vi "CRYRecall Curve Name Replace.vi"(6 "Data type":string, 7 "Setup in":T1={"No.VI"=0, "Category"="", "StepName"="", "Seq setup flattened"="", "Comment"="", "Steps config."=[], "Jump config"=[], "Start"=0.0, "Increment"=0.0, "Name"="Pa", "Unit"="Pa", "Y data"=1, "Y prefix"="", "Y dB ref"=1.0, "Y unit"="", "Repeat State Array"=[]} {"Repeat State Array"."Start" format="%#_5g"; "Y dB ref" format="%.1f"; "Y data" items=["dB", "Lin"]; "Start" format="%#_5g"}, 9 "Step setup In":string, 11 "sOption1":string="SameRemain") -> ()   [LabVIEW 2013]
uses:
  Typedef Control/CRYStep.ctl
  Typedef Control/CRYResult Cluster Array.ctl
  Typedef Control/CRYResult Cluster.ctl
  Typedef Control/CRYData Cluster Array.ctl
  Typedef Control/CRYData Cluster.ctl
  Typedef Control/CRYWaveform Cluster Array.ctl
  Typedef Control/CRYWaveform Cluster.ctl
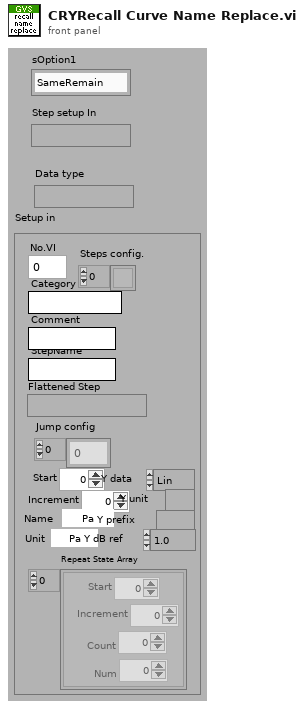
[diagram p1: front panel]
types:
  T1 = typedef "CRYStep.ctl" = cluster{"No.VI":i32, "Category":string, "StepName":string, "Seq setup flattened":string, "Comment":string, "Steps config.":bool[], "Jump config":i32[], "Start":dbl, "Increment":dbl, "Name":string, "Unit":string, "Y data":u16, "Y prefix":string, "Y dB ref":dbl, "Y unit":string, "Repeat State Array":cluster{"Start":dbl, "Increment":dbl, "Count":i32, "Num":i32}[]}
  T2 = typedef "CRYWaveform Cluster Array.ctl" = T3[]
  T3 = typedef "CRYWaveform Cluster.ctl" = cluster{"Waveform":cluster{"X0":dbl, "dX":dbl, "Y":sgl[]}, "X data":u16, "Y data":u16, "Y axis":u16, "X unit":string, "Y unit":string, "Y dB ref":dbl, "display Y":bool, "display X":bool, "Overload?":bool, "Test Info":string, "Step No.":i32, "Name":string, "protected":bool, "Sqc history":string[], "Signal Channel ID":i32, "Plot Settings":cluster{"Color":u32, "Interpolation":u8, "Point Style":u8, "Line Style":u8, "Point Color":u32, "Line Width":u8, "Bar Plot Style":u8, "Fill To":i16}, "AutoProtect":bool}
  T4 = typedef "CRYData Cluster Array.ctl" = T5[]
  T5 = typedef "CRYData Cluster.ctl" = cluster{"Name":string, "Curve":cluster{"x":dbl, "y":dbl, "z":dbl}[], "X data":u16, "Y data":u16, "Z data":u16, "X axis":u16, "Y axis":u16, "Z axis":u16, "X unit":string, "Y unit":string, "Z unit":string, "X dB ref":dbl, "Y dB ref":dbl, "Z dB ref":dbl, "single val":bool, "protected":bool, "display X":bool, "display Y":bool, "display Z":bool, "Test Info":string, "Step No.":i32, "Plot Settings":cluster{"Color":u32, "Interpolation":u8, "Point Style":u8, "Line Style":u8, "Point Color":u32, "Line Width":u8, "Bar Plot Style":u8, "Fill To":i16}, "AutoProtect":bool}
  T6 = typedef "CRYResult Cluster Array.ctl" = T7[]
  T7 = typedef "CRYResult Cluster.ctl" = cluster{"Name":string, "Margin":dbl, "unit":string, "Verdict":bool, "Limit":string, "Max/Min":string, "protected":bool, "Step No.":i32, "Test Info":string, "AutoProtect":bool}
  T8 = cluster{"Start":dbl, "Increment":dbl, "Count":i32, "Num":i32}[]
  T9 = typedef "CRYRecall Cluster.ctl" = cluster{"Name":string, "filepath":string, "all or last":i32, "File Path Mode":u16, "Curve Names":string[], "format string":cluster{"dB Format String out":string, "Lin Format String out":string}, "Template":u16[], "Axis":u16, "*.imp Path":path, "Filepath option":i16, "ML Value":dbl, "user defined":string, "Curves Selected?":bool[], "Help":string, "Tab Value":enum32{"Setting", "Help"}, "Selector":i32, "Use Default":bool}
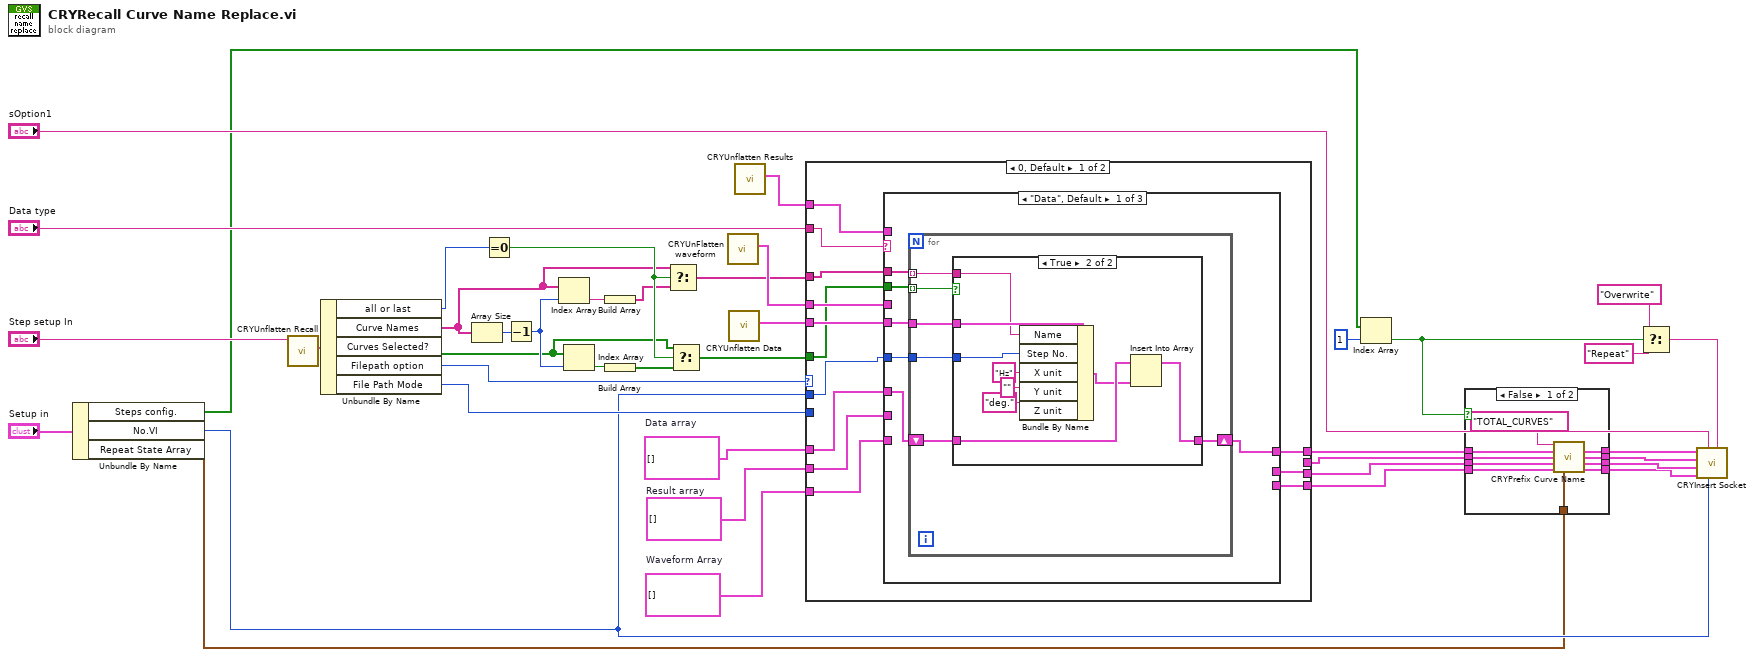
[diagram p0: block diagram]
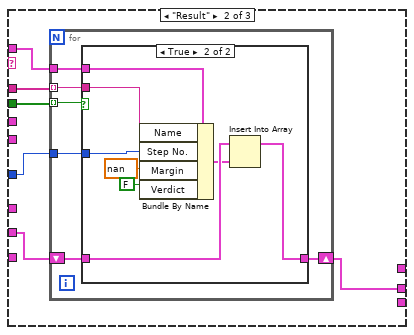
[diagram p4: hidden frame]
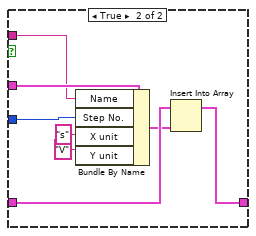
[diagram p7: hidden frame]
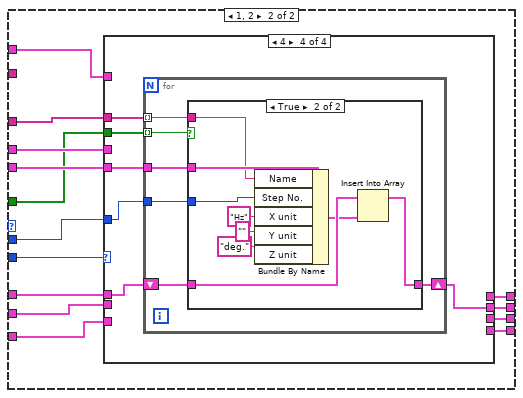
[diagram p8: hidden frame]
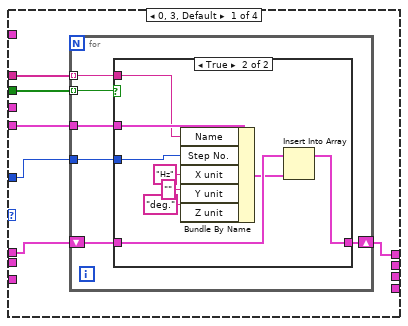
[diagram p9: hidden frame]
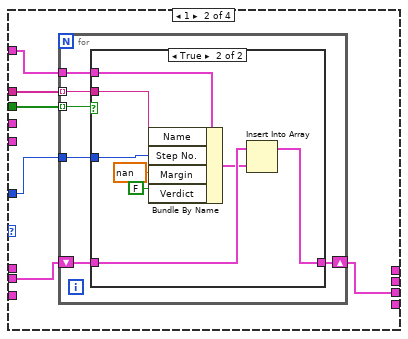
[diagram p11: hidden frame]
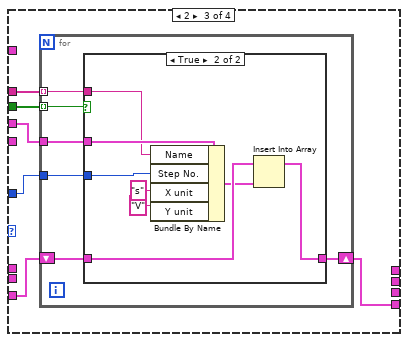
[diagram p13: hidden frame]
diagram:
  w36 = T2 []  # Waveform Array
  w38 = T4 []  # Data array
  w37 = T6 []  # Result array
  n1 = Unbundle By Name("Setup in") -> ("Steps config."=w11:bool[], "No.VI"=w12:i32, "Repeat State Array"=w1:T8)
  n2 = call "CRYUnflatten Recall.vi"("Flatten Recall"="Step setup In") -> ("Recall setup"=w30:T9)  [unwired: 8 in, 2 out]
  n3 = Unbundle By Name(w30) -> ("all or last"=w27:i32, "Curve Names"=w21:string[], "Curves Selected?"=w18:bool[], "Filepath option"=w29:i16, "File Path Mode"=w28:u16)
  n4 = Array Size(array=w21) -> (size(s)=w26:i32)
  n5 = Equal To 0?(x=w27) -> (x = 0?=w22:bool)
  n6 = Decrement(x=w26) -> (x-1=w25:i32)
  n7 = Index Array(array=w21, index=w25) -> (element=w23:string)
  n8 = Index Array(array=w18, index=w25) -> (element=w24:bool)
  n9 = Build Array(w23) -> (w20:string[])
  n10 = Build Array(w24) -> (w19:bool[])
  n11 = Select(t=w21, s=w22, f=w20) -> (s? t:f=w17:string[])
  n12 = Select(t=w18, s=w22, f=w19) -> (s? t:f=w16:bool[])
  n13 = call "CRYUnFlatten waveform.vi"() -> ("Waveform Cluster"=w39:T3)  [unwired: 9 in, 2 out]
  n14 = call "CRYUnflatten Data.vi"() -> ("Datum"=w41:T5)  [unwired: 9 in, 2 out]
  n15 = call "CRYUnflatten Results.vi"() -> ("Result"=w40:T7)  [unwired: 9 in, 2 out]
  n16 = case shown="0, Default" w29 {
    tunnel: w41 -> [w54 w132]
    tunnel: w12 -> [w53 w131]
    tunnel: [w52 w130] -> w10
    tunnel: [_ w129] -> w9
    tunnel: [w50 w128] -> w8
    tunnel: [w49 w127] -> w7
    tunnel: w40 -> [w51 w126]
    tunnel: w39 -> [w48 w125]
    tunnel: w38 -> [w46 w123]
    tunnel: w37 -> [w45 w122]
    tunnel: w36 -> [w47 w124]
    tunnel: w28 -> [_ w121]
    tunnel: w17 -> [w44 w120]
    tunnel: w16 -> [w43 w119]
    tunnel: "Data type" -> [w42 _]
    frame 0, Default {
      n17 = case shown="\"Data\", Default" w42 {
        tunnel: w44 -> [w60 w82 w103]
        tunnel: w43 -> [w59 w81 w102]
        tunnel: w54 -> [w58 _ _]
        tunnel: w53 -> [w57 w79 w100]
        tunnel: w47 -> [_ _ w99]
        tunnel: [w55 _ _] -> w52
        tunnel: w51 -> [_ w80 _]
        tunnel: [_ w78 _] -> w50
        tunnel: [_ _ w98] -> w49
        tunnel: w48 -> [_ _ w101]
        tunnel: w46 -> [w56 _ _]
        tunnel: w45 -> [_ w77 _]
        frame "Data", Default {
          n18 = for {
            tunnel: w60 -> [w66] mode=indexing
            shift-right: [w64] -> w55
            shift-left: w56 -> [w65]
            tunnel: w59 -> [w63] mode=indexing
            tunnel: w58 -> [w62]
            tunnel: w57 -> [w61]
            n19 = case shown="True" w63 {
              tunnel: w66 -> [_ w74]
              tunnel: w65 -> [w67 w70]
              tunnel: [w67 w69] -> w64
              tunnel: w62 -> [_ w76]
              tunnel: w61 -> [_ w75]
              frame False {
              }
              frame True {
                n20 = Bundle By Name(cluster=w76, "Name"=w74, "Step No."=w75, "X unit"="Hz", "Y unit"="", "Z unit"="deg.") -> (w68:T5)
                n21 = Insert Into Array(array=w70, new element=w68) -> (w69:T4)  [unwired: 1 in]
              }
            }
          }
        }
        frame "Result" {
          n22 = for {
            tunnel: w79 -> [w88]
            tunnel: w80 -> [w87]
            tunnel: w82 -> [w85] mode=indexing
            tunnel: w81 -> [w86] mode=indexing
            shift-right: [w83] -> w78
            shift-left: w77 -> [w84]
            n23 = case shown="True" w86 {
              tunnel: w88 -> [_ w97]
              tunnel: w87 -> [_ w96]
              tunnel: w85 -> [_ w95]
              tunnel: w84 -> [w89 w92]
              tunnel: [w89 w91] -> w83
              frame False {
              }
              frame True {
                n24 = Bundle By Name(cluster=w96, "Name"=w95, "Step No."=w97, "Margin"=nan, "Verdict"=FALSE) -> (w90:T7)
                n25 = Insert Into Array(array=w92, new element=w90) -> (w91:T6)  [unwired: 1 in]
              }
            }
          }
        }
        frame "Waveform" {
          n26 = for {
            tunnel: w103 -> [w109] mode=indexing
            shift-right: [w107] -> w98
            shift-left: w99 -> [w108]
            tunnel: w102 -> [w106] mode=indexing
            tunnel: w101 -> [w105]
            tunnel: w100 -> [w104]
            n27 = case shown="False" w106 {
              tunnel: w109 -> [_ w116]
              tunnel: w108 -> [w110 w113]
              tunnel: [w110 w112] -> w107
              tunnel: w105 -> [_ w118]
              tunnel: w104 -> [_ w117]
              frame False {
              }
              frame True {
                n28 = Bundle By Name(cluster=w118, "Name"=w116, "Step No."=w117, "X unit"="s", "Y unit"="V") -> (w111:T3)
                n29 = Insert Into Array(array=w113, new element=w111) -> (w112:T2)  [unwired: 1 in]
              }
            }
          }
        }
      }
    }
    frame 1, 2 {
      n30 = case shown="4" w121 {
        tunnel: w132 -> [w136 _ _ w200]
        tunnel: w131 -> [w135 w159 w178 w199]
        tunnel: w120 -> [w138 w158 w181 w202]
        tunnel: w119 -> [w137 w157 w180 w201]
        tunnel: [w134 _ _ _] -> w130
        tunnel: [_ _ _ w198] -> w129
        tunnel: [_ w156 _ _] -> w128
        tunnel: [_ _ w177 _] -> w127
        tunnel: w126 -> [_ w160 _ _]
        tunnel: w125 -> [_ _ w179 _]
        tunnel: w124 -> [_ _ w176 _]
        tunnel: w123 -> [w133 _ _ w197]
        tunnel: w122 -> [_ w155 _ _]
        frame 0, 3, Default {
          n31 = for {
            tunnel: w138 -> [w144] mode=indexing
            shift-right: [w142] -> w134
            shift-left: w133 -> [w143]
            tunnel: w137 -> [w141] mode=indexing
            tunnel: w136 -> [w140]
            tunnel: w135 -> [w139]
            n32 = case shown="True" w141 {
              tunnel: w144 -> [_ w152]
              tunnel: w143 -> [w145 w148]
              tunnel: [w145 w147] -> w142
              tunnel: w140 -> [_ w154]
              tunnel: w139 -> [_ w153]
              frame False {
              }
              frame True {
                n33 = Bundle By Name(cluster=w154, "Name"=w152, "Step No."=w153, "X unit"="Hz", "Y unit"="", "Z unit"="deg.") -> (w146:T5)
                n34 = Insert Into Array(array=w148, new element=w146) -> (w147:T4)  [unwired: 1 in]
              }
            }
          }
        }
        frame 1 {
          n35 = for {
            tunnel: w159 -> [w166]
            tunnel: w160 -> [w165]
            tunnel: w158 -> [w163] mode=indexing
            tunnel: w157 -> [w164] mode=indexing
            shift-right: [w161] -> w156
            shift-left: w155 -> [w162]
            n36 = case shown="True" w164 {
              tunnel: w166 -> [_ w175]
              tunnel: w165 -> [_ w174]
              tunnel: w163 -> [_ w173]
              tunnel: w162 -> [w167 w170]
              tunnel: [w167 w169] -> w161
              frame False {
              }
              frame True {
                n37 = Bundle By Name(cluster=w174, "Name"=w173, "Step No."=w175, "Margin"=nan, "Verdict"=FALSE) -> (w168:T7)
                n38 = Insert Into Array(array=w170, new element=w168) -> (w169:T6)  [unwired: 1 in]
              }
            }
          }
        }
        frame 2 {
          n39 = for {
            tunnel: w181 -> [w187] mode=indexing
            shift-right: [w185] -> w177
            shift-left: w176 -> [w186]
            tunnel: w180 -> [w184] mode=indexing
            tunnel: w179 -> [w183]
            tunnel: w178 -> [w182]
            n40 = case shown="True" w184 {
              tunnel: w187 -> [_ w194]
              tunnel: w186 -> [w188 w191]
              tunnel: [w188 w190] -> w185
              tunnel: w183 -> [_ w196]
              tunnel: w182 -> [_ w195]
              frame False {
              }
              frame True {
                n41 = Bundle By Name(cluster=w196, "Name"=w194, "Step No."=w195, "X unit"="s", "Y unit"="V") -> (w189:T3)
                n42 = Insert Into Array(array=w191, new element=w189) -> (w190:T2)  [unwired: 1 in]
              }
            }
          }
        }
        frame 4 {
          n43 = for {
            tunnel: w202 -> [w208] mode=indexing
            shift-right: [w206] -> w198
            shift-left: w197 -> [w207]
            tunnel: w201 -> [w205] mode=indexing
            tunnel: w200 -> [w204]
            tunnel: w199 -> [w203]
            n44 = case shown="True" w205 {
              tunnel: w208 -> [_ w216]
              tunnel: w207 -> [w209 w212]
              tunnel: [w209 w211] -> w206
              tunnel: w204 -> [_ w218]
              tunnel: w203 -> [_ w217]
              frame False {
              }
              frame True {
                n45 = Bundle By Name(cluster=w218, "Name"=w216, "Step No."=w217, "X unit"="Hz", "Y unit"="", "Z unit"="deg.") -> (w210:T5)
                n46 = Insert Into Array(array=w212, new element=w210) -> (w211:T4)  [unwired: 1 in]
              }
            }
          }
        }
      }
    }
  }
  n47 = Index Array(array=w11, index=1) -> (element=w2:bool)
  n48 = case shown="False" w2 {
    tunnel: w10 -> [w227 w232]
    tunnel: w9 -> [w226 w231]
    tunnel: w8 -> [w225 w230]
    tunnel: w7 -> [w224 w229]
    tunnel: [w223 w232] -> w6
    tunnel: [w222 w231] -> w5
    tunnel: [w221 w230] -> w4
    tunnel: [w220 w229] -> w3
    tunnel: w1 -> [w219 _]
    frame False {
      n49 = call "CRYPrefix Curve Name.vi"("Type In"="TOTAL_CURVES", "Curves In"=w227, "Values In"=w226, "Results In"=w225, "Waves In"=w224, "Repeat State Array In"=w219) -> ("Curves Out"=w223:T4, "Values Out"=w222:T4, "Results Out"=w221:T6, "Waves Out"=w220:T2)  [unwired: 6 in]
    }
    frame True {
    }
  }
  n50 = Select(t="Overwrite" ("Y unit"), s=w2, f="Repeat") -> (s? t:f=w32:string)
  n51 = call "CRYInsert Socket.vi"("sOption2"=w32, "Step No."=w12, "sOption1"="sOption1", "Waves"=w3, "Results"=w4, "Values"=w5, "Curves"=w6) -> ()  [unwired: 4 in, 1 out]
